vi "ShooterTEST.vi"(5 "WinchCaseIn":dbl, 8 "OutGearPos":dbl=2.1, 9 "InGearPos":dbl=1.5, 10 "Pot":dbl, 11 "Fire":bool) -> (0 "There?":bool, 1 "WinchCase":i32, 3 "Power":dbl)   [LabVIEW 2013]
panel:
  out "Index":i32
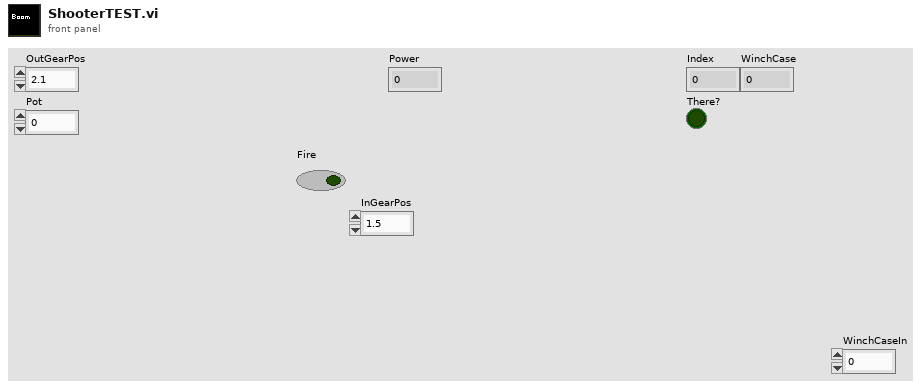
[diagram p1: front panel]
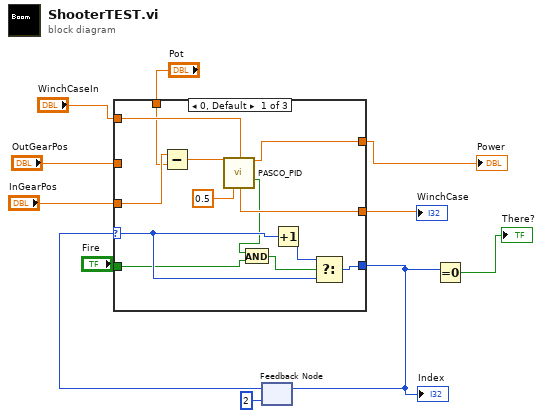
[diagram p0: block diagram]
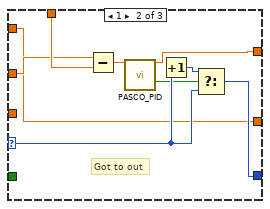
[diagram p2: hidden frame]
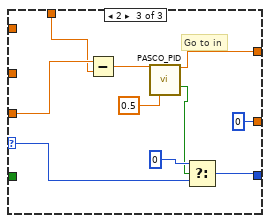
[diagram p3: hidden frame]
diagram:
  n1 = feedback #1(2 ("Numeric")) -> (w9:i32)
  n2 = case shown="0, Default" w9 {
    selector: w9 -> [w21 w30 w40]
    tunnel: [w12 w29 w39] -> w1
    tunnel: "Fire" -> [w13 _ _]
    tunnel: [w23 w32 w42] -> w6
    tunnel: "OutGearPos" -> [_ w25 _]
    tunnel: "InGearPos" -> [w17 _ w37]
    tunnel: "Pot" -> [w16 w26 w36]
    tunnel: [w20 w24 0 ("WinchCase")] -> w3
    tunnel: "WinchCaseIn" -> [w20 w24 _]
    frame 0, Default {
      n3 = Subtract(x=w17, y=w16) -> (x-y=w18:dbl)
      n4 = call "PASCO_PID.vi"("Delta"=w18, "P Gain"=0.5) -> ("Output"=w12:dbl, "IsThere"=w14:bool)  [unwired: 12 in]
      n5 = And(x=w14, y=w13) -> (x .and. y?=w15:bool)
      n6 = Increment(x=w21) -> (x+1=w22:i32)
      n7 = Select(t=w22, s=w15, f=w21) -> (s? t:f=w23:i32)
    }
    frame 1 {
      # "Got to out"
      n8 = Subtract(x=w25, y=w26) -> (x-y=w27:dbl)
      n9 = call "PASCO_PID.vi"("Delta"=w27) -> ("Output"=w29:dbl, "IsThere"=w28:bool)  [unwired: 13 in]
      n10 = Increment(x=w30) -> (x+1=w31:i32)
      n11 = Select(t=w31, s=w28, f=w30) -> (s? t:f=w32:i32)
    }
    frame 2 {
      # "Go to in"
      n12 = Subtract(x=w37, y=w36) -> (x-y=w35:dbl)
      n13 = call "PASCO_PID.vi"("Delta"=w35, "P Gain"=0.5) -> ("Output"=w39:dbl, "IsThere"=w38:bool)  [unwired: 12 in]
      n14 = Select(t=0, s=w38, f=w40) -> (s? t:f=w42:i32)
    }
  }
  "Power" <- w1
  "Index" <- w6
  "WinchCase" <- w3
  n15 = feedback-in #1(w6) -> ()
  n16 = Equal To 0?(x=w6) -> (x = 0?=→"There?":bool)
